vi "SetPosition.vi"(8 "error in (no error)":errorcluster, 10 "position":cluster{"left":u32, "top":u32}, 11 "separator item in":refnum<class "separator item.lvclass">) -> (0 "error out":errorcluster, 3 "separator item out":refnum<class "separator item.lvclass">)   [LabVIEW 2009, in "separator item.lvclass"]
uses:
  separator item.lvclass
  separator item.lvclass/separator item.ctl
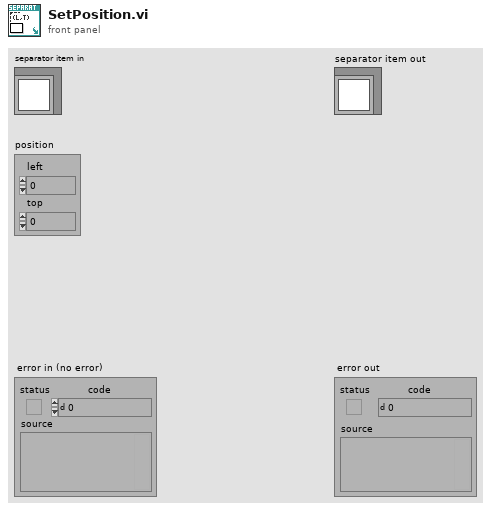
[diagram p1: front panel]
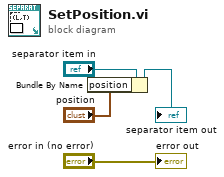
[diagram p0: block diagram]
diagram:
  n1 = Bundle By Name(cluster="separator item in", "position"="position") -> (→"separator item out":refnum<class "separator item.lvclass">)
  "error out" <- "error in (no error)"
